vi "Pfeiffer Vacuum Handheld Vacuum Gauge.vi"(8 "error in (no error)":errorcluster, 9 "Handheld Gauge Data-Cluster":T1={"Parameter"=0, "Parameter\nread only<->describe"=FALSE, "Correction facktor\n(0,20 - 8,00) "=1.0, "Physical units"=0} {"Physical units" items=["mbar", "Pa", "Atm", "Torr", "hPa "]; "Correction facktor\n(0,20 - 8,00)" min=0.2 max=8 step=0.01 format="%.2f"; "Parameter" items=[" Pressure (read only) [mbar]", " Correction factor Pirani", " Actual error code (read only)", " Software version Transmitter  (read only)", " Unit type Transmitter (read only)", " Physical units"]}, 10 "Adress of unit":u16=1 min=1 max=999 step=1, 11 "VISA session in":refnum<visa-resource-name>) -> (0 "error out":errorcluster, 3 "response (data)":string)   [LabVIEW 2016]
doc: "This VI is an example of how to use the Pfeiffer Vacuum subVIs programmatically. This VI first initializes the instrument, takes measurements, then closes the instrument."
uses:
  Public/Handheld Gauge/Handheld Gauge Data - Cluster.ctl
  Pfeiffer Vacuum.lvlib
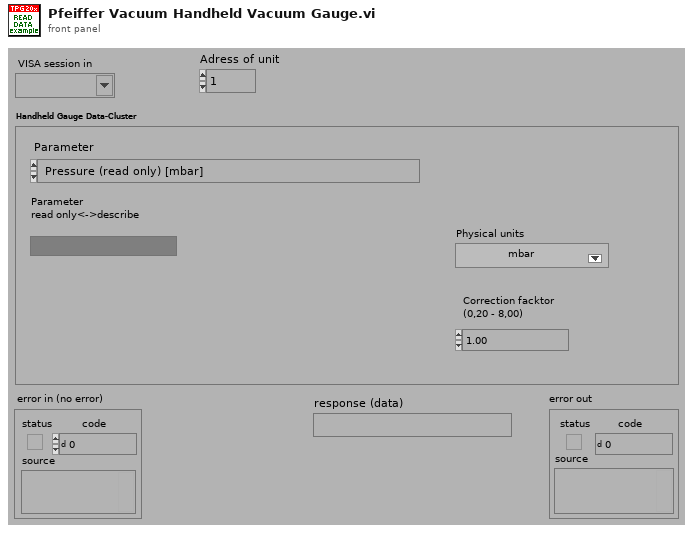
[diagram p1: front panel]
types:
  T1 = typedef "Pfeiffer Vacuum.lvlib/Handheld Gauge Data - Cluster.ctl" = cluster{"Parameter":u16, "Parameter\nread only<->describe":bool, "Correction facktor\n(0,20 - 8,00) ":sgl, "Physical units":u16}
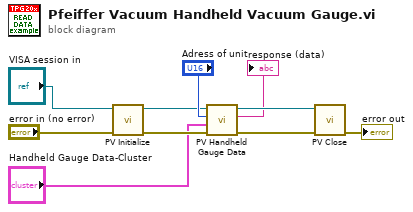
[diagram p0: block diagram]
diagram:
  n1 = call "PV Initialize.vi"("error in (no error)"="error in (no error)", "VISA session in"="VISA session in") -> ("error out"=w4:errorcluster, "VISA session out"=w3:refnum<visa-resource-name>)  [unwired: 8 in]
  n2 = call "PV Handheld Gauge Data.vi"("error in (no error)"=w4, "Handheld Gauge Data-Cluster"="Handheld Gauge Data-Cluster", "Adress of unit"="Adress of unit", "VISA session"=w3) -> ("error out"=w10:errorcluster, "response (data)"=→"response (data)":string, "dup VISA session"=w9:refnum<visa-resource-name>)  [unwired: 5 in]
  n3 = call "PV Close.vi"("VISA session"=w9, "error in (no error)"=w10) -> ("error out"=→"error out":errorcluster)  [unwired: 13 in]
